vi "DecodeCommand.vi"(1 "element":u8[](array[numeric]), 5 "error in (no error)":errorcluster) -> (14 "Command":T1, 19 "error out":errorcluster)   [LabVIEW 2023, in "Referee.lvclass"]
uses:
  Referee.lvclass
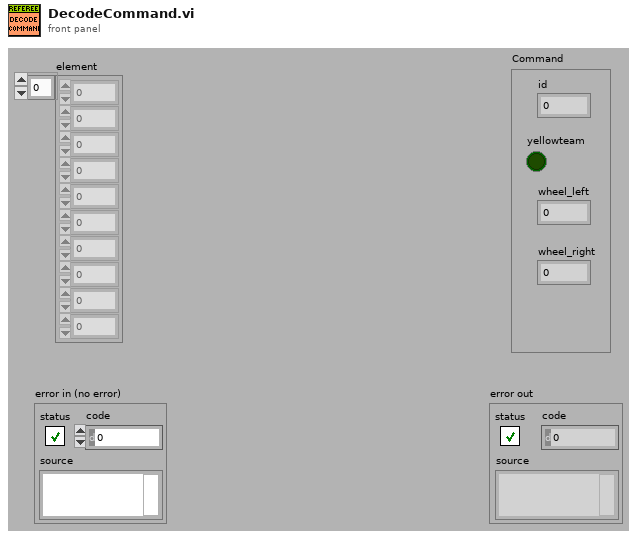
[diagram p1: front panel]
types:
  T1 = cluster{"id":dbl, "yellowteam":bool, "wheel_left":dbl, "wheel_right":dbl}
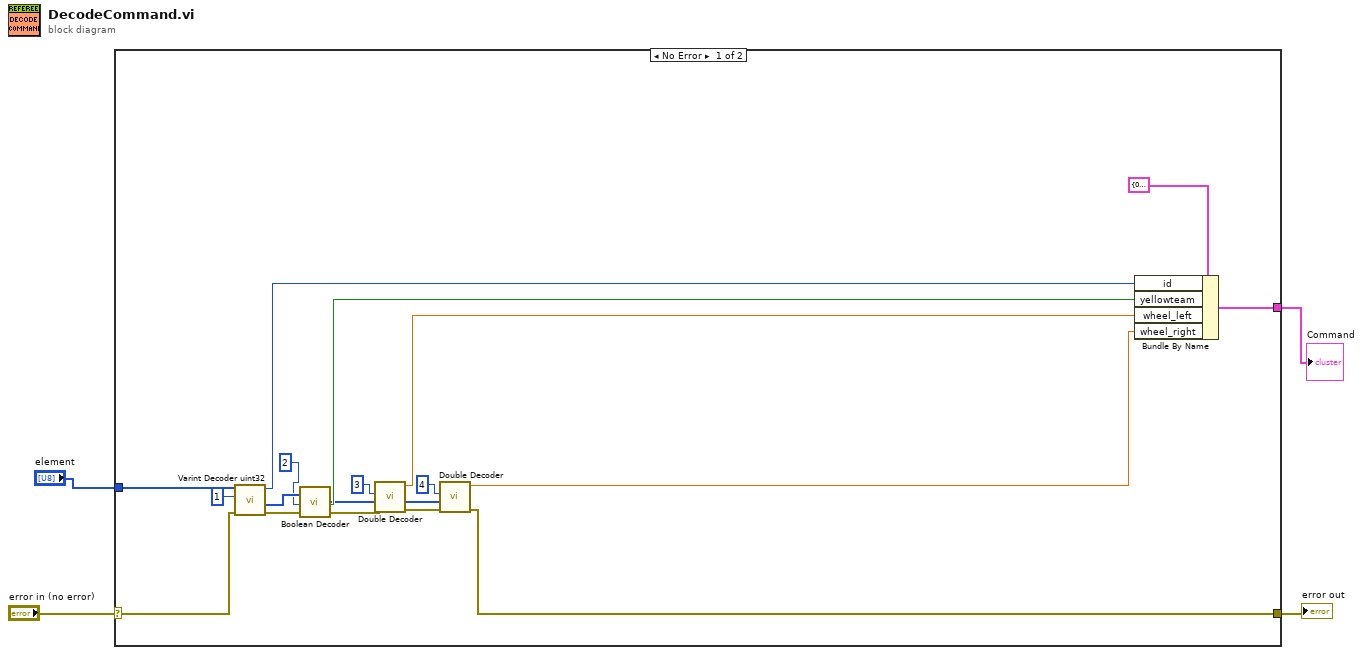
[diagram p0: block diagram]
diagram:
  n1 = case shown="No Error" "error in (no error)" {
    selector: "error in (no error)" -> [w9 w24]
    tunnel: [w10 w24] -> w3
    tunnel: "element" -> [w20 _]
    tunnel: [w22 _] -> w1
    frame No Error {
      n2 = call "Varint Decoder uint32.vi"("error in (no error)"=w9, "Array"=w20, "Key"=1) -> ("error out"=w8:errorcluster, "array w/ subset deleted"=w7:u8[], "Varint"=w19:u32)  [unwired: 5 in, 1 out]
      n3 = call "Boolean Decoder.vi"("array"=w7, "Key"=2, "error in (no error)"=w8) -> ("array w/ subset deleted"=w5:u8[], "Bool"=w13:bool, "error out"=w12:errorcluster)  [unwired: 14 in]
      n4 = call "Double Decoder.vi"("error in (no error)"=w12, "Array"=w5, "Key"=3) -> ("error out"=w11:errorcluster, "array w/ subset deleted"=w16:u8[], "Double"=w15:dbl)  [unwired: 5 in, 1 out]
      n5 = call "Double Decoder.vi"("error in (no error)"=w11, "Array"=w16, "Key"=4) -> ("error out"=w10:errorcluster, "Double"=w14:dbl)  [unwired: 5 in, 2 out]
      n6 = Bundle By Name(cluster=T1 {"id"=0.0, "yellowteam"=FALSE, "wheel_left"=0.0, "wheel_right"=0.0} ("Command"), "id"=w19, "yellowteam"=w13, "wheel_left"=w15, "wheel_right"=w14) -> (w22:T1)
    }
    frame Error {
    }
  }
  "error out" <- w3
  "Command" <- w1
